vi "Dot Tracking.vi"(0 "X Parameters":T2={"Number of X Steps"=200, "Max X (V)"=1.0, "Min X (V)"=-1.0}, 1 "Y Parameters":T1={"Number of Y Steps"=200, "Max Y (V)"=1.0, "Min Y (V)"=-1.0}, 3 "RS232 settings":cluster{"Portnumber":i32, "Baudrate":u16}={"Portnumber"=12, "Baudrate"=5} {"Portnumber" items=["COM1", "COM2", "COM3", "COM4", "COM5", "COM6", "COM7", "COM8", "COM9", "COM10", "COM11", "COM12", "COM13", "COM14", "COM15", "COM16", "COM17", "COM18", "COM19", "COM20", "COM21", "COM22", "COM23", "COM24", "COM25", "COM26", "COM27", "COM28", "COM29", "COM30"]; "Baudrate" items=["9600", "14400", "19200", "38400", "57600", "115200"]}, 5 "X Pos":dbl=192.0, 9 "Y pos":dbl=35.0, 11 "Z Pos":dbl=52.1, 14 "Z-track?":bool=TRUE) -> (4 "X Position":dbl, 6 "Y Position":dbl, 8 "Y Gauss Amplitude":dbl, 10 "Z Position":dbl, 12 "Cross Section X":dbl[](graph), 13 "Cross Section Y":dbl[](graph), 15 "Gave up?":bool)   [LabVIEW 2011]
panel:
  out "Center Y":dbl
  out "Center X":dbl
  in  "stop":bool
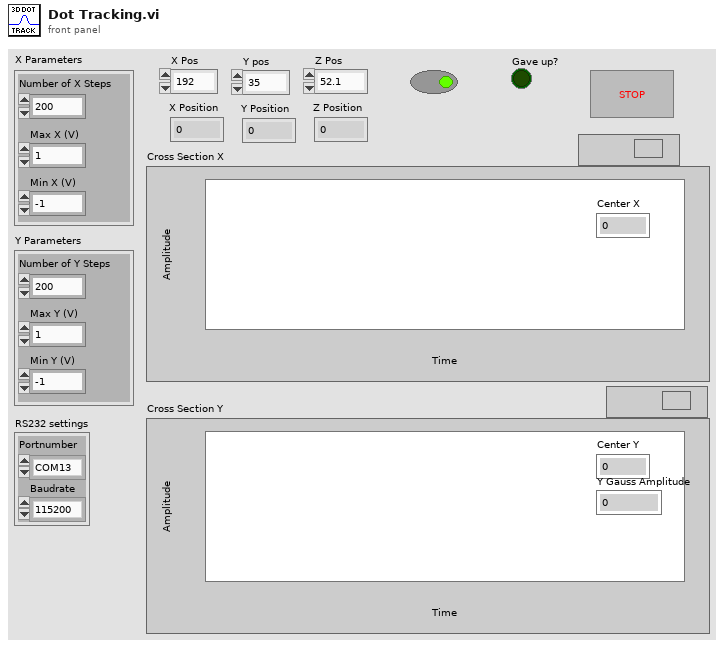
[diagram p1: front panel]
types:
  T1 = cluster{"Number of Y Steps":i32, "Max Y (V)":dbl, "Min Y (V)":dbl}
  T2 = cluster{"Number of X Steps":i32, "Max X (V)":dbl, "Min X (V)":dbl}
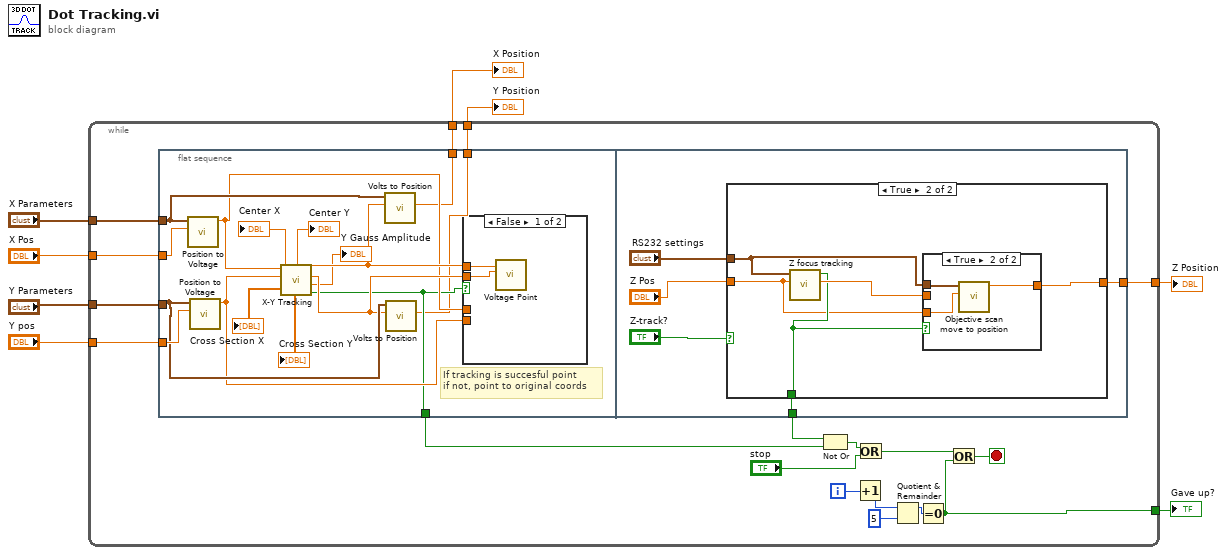
[diagram p0: block diagram]
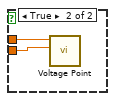
[diagram p2: hidden frame]
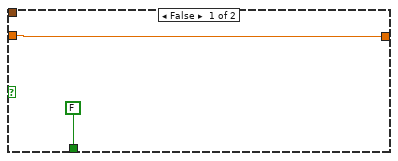
[diagram p3: hidden frame]
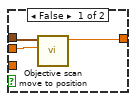
[diagram p4: hidden frame]
diagram:
  n1 = while {
    tunnel: "X Pos" -> [w26]
    tunnel: "Y Parameters" -> [w25]
    tunnel: "Y pos" -> [w24]
    tunnel: [w13] -> w4
    tunnel: "X Parameters" -> [w15]
    tunnel: [w11] -> w3
    tunnel: [w10] -> w1
    tunnel: [w9] -> w2
    i -> [w17]
    stop <- w16 stop-if-true
    n2 = flat-sequence {
      tunnel: w26 -> [w41]
      tunnel: w25 -> [w35]
      tunnel: w24 -> [w42]
      tunnel: w15 -> [w36]
      tunnel: [w30] -> w12
      tunnel: [w29] -> w10
      tunnel: [w28] -> w9
      tunnel: [w51] -> w23
      tunnel: [w47] -> w11
      frame #0 {
        # "If tracking is succesful point \nif not, point to original coords"
        n3 = call "Position to Voltage.vi"("X Pos"=w41, "X Parameters"=w36) -> ("Voltage"=w32:dbl)  [unwired: 9 in]
        n4 = call "Position to Voltage.vi"("X Pos"=w42, "X Parameters"=w35) -> ("Voltage"=w31:dbl)  [unwired: 9 in]
        n5 = call "X-Y Tracking.vi"("Y Voltage"=w31, "X Voltage"=w32) -> ("gave up?"=w30:bool, "Y Gauss Amplitude"=→"Y Gauss Amplitude":dbl, "Y centered Voltage"=w33:dbl, "X Centered Voltage"=w34:dbl, "Cross Section Y"=→"Cross Section Y":dbl[], "Center Y"=→"Center Y":dbl, "Cross Section X"=→"Cross Section X":dbl[], "Center X"=→"Center X":dbl)  [unwired: 2 in]
        n6 = call "Volts to Position.vi"("X Voltage"=w34, "X Parameters"=w36) -> ("Result"=w29:dbl)  [unwired: 9 in]
        n7 = call "Volts to Position.vi"("X Voltage"=w33, "X Parameters"=w35) -> ("Result"=w28:dbl)  [unwired: 9 in]
        n8 = case shown="False" w30 {
          tunnel: w34 -> [w44 _]
          tunnel: w33 -> [w43 _]
          tunnel: w32 -> [_ w46]
          tunnel: w31 -> [_ w45]
          frame False {
            n9 = call "Voltage Point.vi"("Y Voltage"=w43, "X Voltage"=w44) -> ()  [unwired: 9 in, 1 out]
          }
          frame True {
            n10 = call "Voltage Point.vi"("Y Voltage"=w45, "X Voltage"=w46) -> ()  [unwired: 9 in, 1 out]
          }
        }
      }
      frame #1 {
        n11 = case shown="True" "Z-track?" {
          tunnel: [FALSE ("give up?") w57] -> w51
          tunnel: "Z Pos" -> [w52 w56]
          tunnel: "RS232 settings" -> [_ w55]
          tunnel: [w52 w54] -> w47
          frame False {
          }
          frame True {
            n12 = call "Z focus tracking.vi"("Position"=w56, "RS232 settings"=w55) -> ("center"=w58:dbl, "give up?"=w57:bool)  [unwired: 6 in, 1 out]
            n13 = case shown="True" w57 {
              tunnel: w58 -> [w61 _]
              tunnel: [w60 w64] -> w54
              tunnel: w55 -> [w59 w62]
              tunnel: w56 -> [_ w63]
              frame False {
                n14 = call "Objective scan move to position.vi"("Z position"=w61, "RS232 settings"=w59) -> ("Z Position 2"=w60:dbl)  [unwired: 9 in]
              }
              frame True {
                n15 = call "Objective scan move to position.vi"("Z position"=w63, "RS232 settings"=w62) -> ("Z Position 2"=w64:dbl)  [unwired: 9 in]
              }
            }
          }
        }
      }
    }
    n16 = Not Or(1:w12, 2:w23) -> (0:w22:bool)
    n17 = Increment(x=w17) -> (x+1=w20:i32)
    n18 = Or(x=w22, y="stop") -> (x .or. y?=w14:bool)
    n19 = Quotient & Remainder(x=w20, y=5) -> (x-y*floor(x/y)=w19:i32)  [unwired: 1 out]
    n20 = Equal To 0?(x=w19) -> (x = 0?=w13:bool)
    n21 = Or(x=w14, y=w13) -> (x .or. y?=w16:bool)
  }
  "X Position" <- w1
  "Y Position" <- w2
  "Z Position" <- w3
  "Gave up?" <- w4
